vi "Configure_Gill.vi"(0 "Analogue O/P Config":u16(ring) items=["0 to 5 volt", "+/-2.5 Volt", "4-20mA"], 1 "ORIGINAL Address":u8=66 min=65 max=90, 2 "NEW Address":u8=66 min=65 max=90, 5 "Analogue O/P Scale":u16(ring) items=["10m/s", "20m/s", "30m/s", "40m/s", "50m/s", "60m/s", "70m/s"], 7 "Averaging Time":u16(ring)=3 items=["OFF", "3 seconds", "5 seconds", "10 seconds"], 9 "Samples/sec":u16(ring) items=["1 sample/sec", "4 samples/sec"], 12 "Port Name":string="Edge0164-P2") -> ()   [LabVIEW 2014]
panel:
  out "Read":string[](array[string])
  out "Write":string[](array[string])
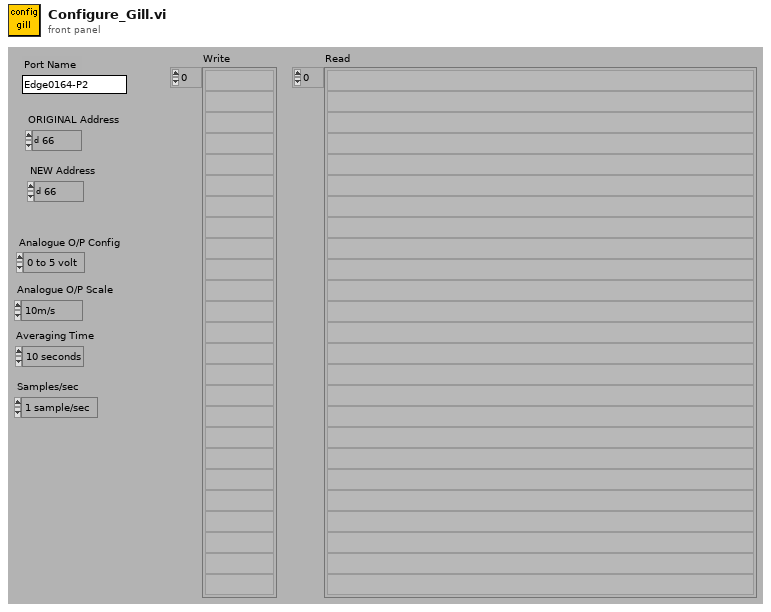
[diagram p1: front panel]
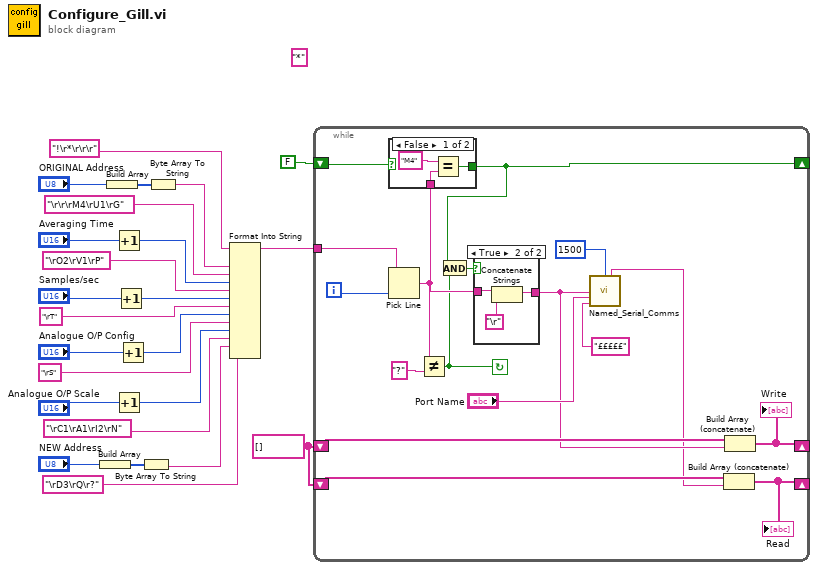
[diagram p0: block diagram]
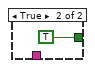
[diagram p2: hidden frame]
diagram:
  w1 = string[] []
  (unwired) "*"
  n1 = Build Array("NEW Address") -> (w14:u8[])
  n2 = Build Array("ORIGINAL Address") -> (w24:u8[])
  n3 = Increment(x="Averaging Time") -> (x+1=w18:u16)
  n4 = Increment(x="Analogue O/P Scale") -> (x+1=w5:u16)
  n5 = Increment(x="Samples/sec") -> (x+1=w16:u16)
  n6 = Increment(x="Analogue O/P Config") -> (x+1=w8:u16)
  n7 = Byte Array To String(unsigned byte array=w14) -> (string=w3:string)
  n8 = Byte Array To String(unsigned byte array=w24) -> (string=w20:string)
  n9 = Format Into String(initial string="!\r*\r\r\r", w20, "\r\r\rM4\rU1\rG", w18, "\rO2\rV1\rP", w16, "\rT", w8, "\rS", w5, "\rC1\rA1\rI2\rN", w3, "\rD3\rQ\r?") -> (resulting string=w21:string)  [unwired: 2 in, 1 out]
  n10 = while {
    shift-left: FALSE -> [w37]
    shift-right: [w36] -> _
    tunnel: w21 -> [w41]
    shift-right: [w31] -> _
    shift-left: w1 -> [w32]
    shift-right: [w27] -> _
    shift-left: w1 -> [w26]
    i -> [w40]
    stop <- w34 continue-if-true
    n11 = Pick Line(multi-line string=w41, line index=w40) -> (output string=w38:string)  [unwired: 1 out]
    n12 = case shown="False" w37 {
      tunnel: w38 -> [w43 _]
      tunnel: [w42 TRUE] -> w36
      frame False {
        n13 = Equal?(x="M4", y=w43) -> (x = y?=w42:bool)
      }
      frame True {
      }
    }
    n14 = Not Equal?(x=w38, y="?") -> (x != y?=w34:bool)
    n15 = And(x=w36, y=w34) -> (x .and. y?=w35:bool)
    n16 = case shown="True" w35 {
      tunnel: [w46 w49] -> w28
      tunnel: w38 -> [w46 w48]
      frame False {
      }
      frame True {
        n17 = Concatenate Strings(w48, "\r") -> (w49:string)
      }
    }
    n18 = call "Named_Serial_Comms.vi"("Write String"=w28, "Timeout/ms"=u32 1500, "Port Name"="Port Name", "Term Grep"="£££££") -> ("Read"=w25:string)  [unwired: 5 in, 6 out]
    n19 = Build Array (concatenate)(w26, w25) -> (w27:string[])
    "Read" <- w27
    n20 = Build Array (concatenate)(w32, w28) -> (w31:string[])
    "Write" <- w31
  }
